vi "系统设置全局变量.vi"() -> ()   [LabVIEW 2016]
panel:
  in  "仪器自动断电":T1={"开关"=enum."关闭", "偏置"=0, "间隔"=30} {"间隔" format="%02.0f"; "偏置" format="%02.0f"}
  in  "title":string="水质在线自动监测系统"
  in  "通电":bool
  in  "数据库类型":T2
  in  "运行周期":T3={"运行模式"=enum."维护模式", "质控频次"=enum."关闭", "空白核查时间"=2, "跨度核查时间"=6, "多参数测试间隔"=30, "湿化学测试间隔"=240} {"跨度核查时间" items=["00H", "01H", "02H", "03H", "04H", "05H", "06H", "07H", "08H", "09H", "10H", "11H", "12H", "13H", "14H", "15H", "16H", "17H", "18H", "19H", "20H", "21H", "22H", "23H", "关闭"]; "空白核查时间" items=["00H", "01H", "02H", "03H", "04H", "05H", "06H", "07H", "08H", "09H", "10H", "11H", "12H", "13H", "14H", "15H", "16H", "17H", "18H", "19H", "20H", "21H", "22H", "23H", "关闭"]}
  in  "模块启用":cluster{"原位多参数":bool, "集成多参数":bool, "营养盐":bool}={"原位多参数"=TRUE, "集成多参数"=TRUE, "营养盐"=TRUE}
  in  "站点系列号":string
  in  "站点名称":string
  in  "系统重启设置":T4 {"分" max=59 format="%02.0f"; "时" max=23 format="%02.0f"}
  # "开关："
  # "起始（分）："
  # "间隔（分）："
  # "多参数测试间隔："
  # "湿化学测试间隔："
  # "质控频次："
  # "运行模式："
  # "跨度核查时间："
  # "零点核查时间："
  # "频次："
  # "时间："
  # "："
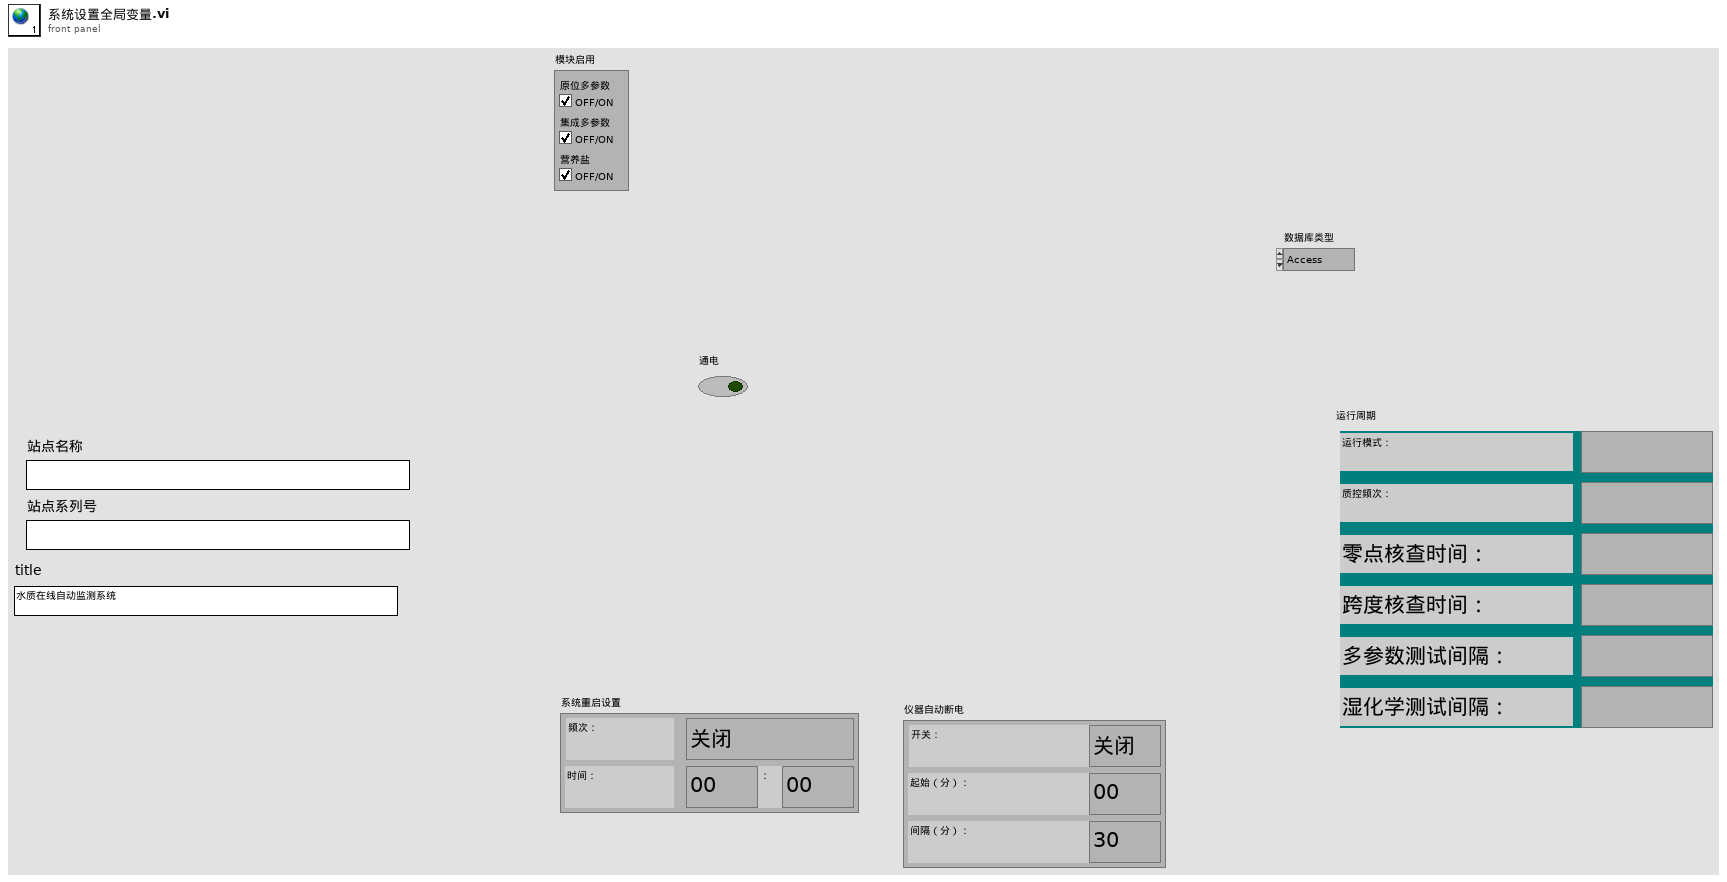
[diagram p1: front panel]
types:
  T1 = cluster{"开关":enum16{"关闭", "打开"}, "偏置":u16, "间隔":u16}
  T2 = typedef "数据库类型.ctl" = enum16{"Access", "SQLite"}
  T3 = cluster{"运行模式":enum16{"维护模式", "常规模式", "应急模式", "质控模式"}, "质控频次":enum16{"关闭", "每天", "星期一", "星期二", "星期三", "星期四", "星期五", "星期六", "星期日"}, "空白核查时间":u16, "跨度核查时间":u16, "多参数测试间隔":u16, "湿化学测试间隔":u16}
  T4 = cluster{"频次":enum16{"关闭", "每天", "星期一", "星期二", "星期三", "星期四", "星期五", "星期六", "星期日"}, "时":u16, "分":u16}
diagram:
